vi "UpdateRequestDescription.vi"(8 "error in":errorcluster, 9 "Description":string, 10 "RequestID":string) -> (0 "error out":errorcluster)   [LabVIEW 2015, in "DatabaseApi.lvlib"]
uses:
  DatabaseApi.lvlib
  TypeDef/Request/RequestsTableColumnNamesRing.ctl
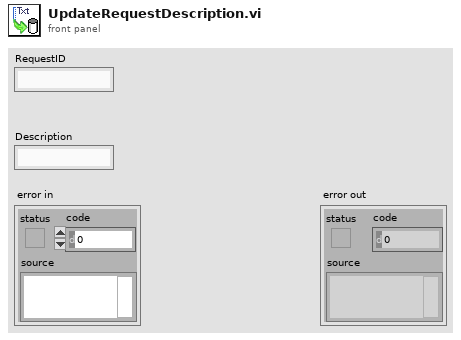
[diagram p1: front panel]
types:
  T1 = typedef "DatabaseApi.lvlib/RequestsTableColumnNamesRing.ctl" = enum16{"RequestID", "PersonnelType", "StartTime", "StartName", "AckTime", "AckName", "FulfilledTime", "FulfilledName", "Description", "Room Number", "Request Type"}
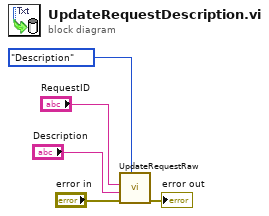
[diagram p0: block diagram]
diagram:
  n1 = call "UpdateRequestRaw.vi"("Data to update"=RequestsTableColumnNamesRing."Description", "error in"="error in", "data"="Description", "RequestID"="RequestID") -> ("error out"=→"error out":errorcluster)  [unwired: 7 in]
